vi "OAT Envelope Detection (Waveform Output, N Channels).vi"(0 "scaled signals [EU]":waveform(dbl)[](array[waveform]), 1 "reset? (F)":bool, 9 "band specification":T1={"center frequency [Hz]"=4800.0, "span [Hz]"=2000.0}, 11 "error in (no error)":errorcluster) -> (4 "envelope signals [EU]":waveform(dbl)[](array[waveform]), 15 "error out":errorcluster)   [LabVIEW 2017, in "SoundVib_FaultAnalysis.lvlib"]
doc: "Extracts the modulating signal, or envelope signal, from an amplitude-modulated signal. You can use the envelope detection technique to identify the mechanical faults that have amplitude-modulating effect on the vibration signal of a machine. Wire data to the <B>scaled signal [EU]</B> input to determine the polymorphic instance to use or manually select the instance."
uses:
  <vilib>/addons/Sound and Vibration/Order Analysis/Fault Analysis/SoundVib_FaultAnalysis.lvlib
  <vilib>/addons/_NISVFA/_Shared subVIs/Common/svc_Check for Waveform Parameter Continuity (no state).vi
  <vilib>/addons/Sound and Vibration/Order Analysis/Resample Order Tracking/SubVIs/oa_Calculate CIC Decimation Filter Coefficients.vi
  <vilib>/addons/Sound and Vibration/Order Analysis/Fault Analysis/SubVIs/sv_Compute Shift and Low Pass Filter with IC.vi
  <vilib>/addons/_NISVFA/_Shared subVIs/Common/svc_Get SV Channel Info.vi
  <vilib>/addons/Sound and Vibration/Order Analysis/Resample Order Tracking/SubVIs/OAT Frequency Shift (Mixer).vi
  <vilib>/addons/Sound and Vibration/Order Analysis/Resample Order Tracking/SubVIs/oa_Decimation with CIC and Compensation Filter.vi
  <vilib>/addons/Sound and Vibration/Order Analysis/Fault Analysis/SubVIs/oa_Demodulation Initial States (1 Channel).vi
  <vilib>/addons/Sound and Vibration/Order Analysis/Adv Resampling/OAT Single Stage Decimation with IC.vi
  <vilib>/addons/Sound and Vibration/Order Analysis/Resample Order Tracking/SubVIs/OAT CIC Decimation.vi
  <vilib>/addons/Sound and Vibration/Order Analysis/Resample Order Tracking/SubVIs/oa_Interpolate Zeros Between Samples.vi
  <vilib>/addons/Sound and Vibration/Order Analysis/Resample Order Tracking/SubVIs/oa_Calculate Delay of CIC Decimation Interpolation Filter.vi
  <vilib>/addons/Sound and Vibration/Order Analysis/Resample Order Tracking/SubVIs/oa_Create CIC Compensation Filter.vi
  <vilib>/addons/Sound and Vibration/Order Analysis/Resample Order Tracking/SubVIs/oa_Create CIC LP Truncation Filter.vi
  <vilib>/addons/_NISVFA/_Shared subVIs/Common/svc_Engineering Units to Unit Label.vi
  <vilib>/addons/_NISVFA/_Shared subVIs/Common/svc_Unit Label to Engineering Units.vi
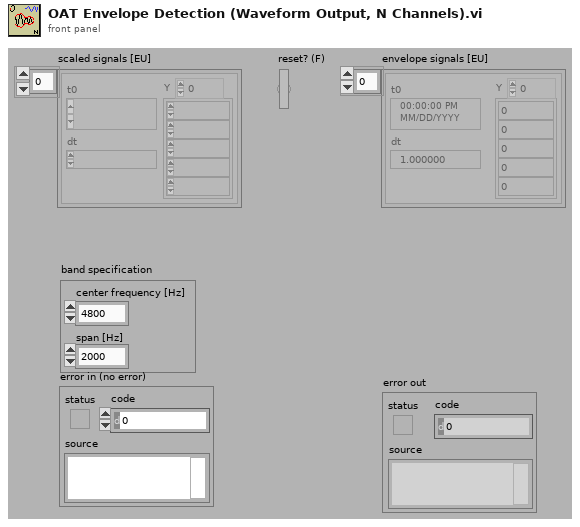
[diagram p1: front panel]
types:
  T1 = cluster{"center frequency [Hz]":dbl, "span [Hz]":dbl}
  T2 = cluster{"dt equal":bool, "array length equal":bool, "number channels change":bool}
  T3 = cluster{"dt":bool, "t0 continuity":bool, "array length":bool, "channel info":bool, "name":bool}
  T4 = typedef "OAT Decimation Filter.ctl" = cluster{"coefficients":dbl[], "factor":i32}
  T5 = cluster{"filter settings":cluster{"CIC Settings":cluster{"Numeric":i32, i32, i32}, "filters":T4[], "delay":i32, "interpolation factor":i32}, "filter states":cluster{"t0":dbl, "phase":dbl, "real filter state":cluster{cluster{dbl[]}, cluster{dbl[]}[]}, "imaginary filter state":cluster{cluster{dbl[]}, cluster{dbl[]}[]}, "delay":i32}[], "reset pending":bool}
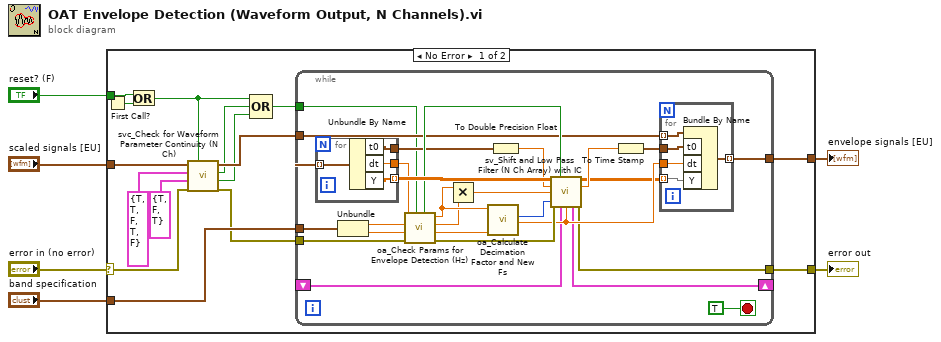
[diagram p0: block diagram]
diagram:
  n1 = case shown="No Error" "error in (no error)" {
    selector: "error in (no error)" -> [w14 w57]
    tunnel: [w17 w57] -> w5
    tunnel: "band specification" -> [w19 _]
    tunnel: "scaled signals [EU]" -> [w16 _]
    tunnel: "reset? (F)" -> [w21 _]
    tunnel: [w18 _] -> w1
    frame No Error {
      n2 = First Call?() -> (First Call?: T/F=w20:bool)
      n3 = Or(x=w21, y=w20) -> (x .or. y?=w10:bool)
      n4 = call <vilib>:"svc_Check for Waveform Parameter Continuity (N Ch).vi"("restart averaging (F)"=w10, "error in (no error)"=w14, "checks for multichannel parameters"=T2 {"dt equal"=TRUE, "array length equal"=FALSE, "number channels change"=TRUE}, "checks for channel parameter change"=T3 {"dt"=TRUE, "t0 continuity"=TRUE, "array length"=FALSE, "channel info"=TRUE, "name"=FALSE}, "scaled signal(s)"=w16) -> ("error out"=w7:errorcluster, "multichannel parameter changed"=w11:bool, "waveform parameter changed"=w12:bool, "dup scaled signal(s)"=w15:waveform(dbl)[])  [unwired: 3 out]
      n5 = Compound Arithmetic op=OR(w10, w12, w11) -> (w13:bool)
      n6 = while {
        tunnel: w19 -> [w47]
        tunnel: [w32] -> w18
        tunnel: [w31] -> w17
        tunnel: w15 -> [w28]
        tunnel: w13 -> [w27]
        tunnel: w7 -> [w26]
        shift-right: [w25] -> _
        shift-left: _ -> [w24]
        stop <- TRUE stop-if-true
        n7 = for {
          tunnel: w28 -> [w56] mode=indexing
          tunnel: [w55] -> w44 mode=indexing
          tunnel: [w54] -> w38
          tunnel: [w53] -> w40
          n8 = Unbundle By Name(w56) -> ("t0"=w54:timestamp, "dt"=w53:dbl, "Y"=w55:dbl[])
        }
        n9 = Unbundle(w47) -> ("center frequency [Hz]"=w45:dbl, "span [Hz]"=w46:dbl)
        n10 = call <vilib>:"oa_Check Params for Envelope Detection (Hz).vi"("reset"=w27, "error in (no error)"=w26, "span"=w46, "center"=w45, "dt"=w40) -> ("error out"=w36:errorcluster, "span out"=w42:dbl, "center out"=w29:dbl, "dt out"=w30:dbl, "reset out"=w43:bool)  [unwired: 1 in, 1 out]
        n11 = Multiply(x=w30, y=w29) -> (x*y=w39:dbl)
        n12 = call <vilib>:"oa_Calculate Decimation Factor and New Fs.vi"("span"=w42, "dt"=w30) -> ("new dt"=w35:dbl, "decimation factor"=w41:i32)  [unwired: 8 in]
        n13 = To Double Precision Float(number=w38) -> (double precision float=w37:dbl)
        n14 = call <vilib>:"sv_Shift and Low Pass Filter (N Ch Array) with IC.vi"("input signals"=w44, "reset? (F)"=w43, "t0"=w37, "center"=w39, "decimation factor"=w41, "error in (no error)"=w36, "initial conditions"=w24, "new dt"=w35) -> ("enveloped signals"=w22:dbl[][], "t0 out"=w34:dbl, "final conditions"=w25:T5, "error out"=w31:errorcluster)  [unwired: 4 in]
        n15 = To Time Stamp(1:w34) -> (0:w33:timestamp)
        n16 = for {
          tunnel: w22 -> [w52] mode=indexing
          tunnel: w35 -> [w51]
          tunnel: w33 -> [w50]
          tunnel: [w49] -> w32 mode=indexing
          tunnel: w28 -> [w48] mode=indexing
          n17 = Bundle By Name(cluster=w48, "t0"=w50, "dt"=w51, "Y"=w52) -> (w49:waveform(dbl))
        }
      }
    }
    frame Error {
    }
  }
  "error out" <- w5
  "envelope signals [EU]" <- w1
